vi "write_single_line.vi"(3 "error in (no error)":errorcluster, 4 "First line?":bool, 5 "Data":dbl, 6 "refnum in":refnum<file>) -> (0 "error out":errorcluster, 1 "String":string, 2 "refnum out":refnum<file>)   [LabVIEW 2015]
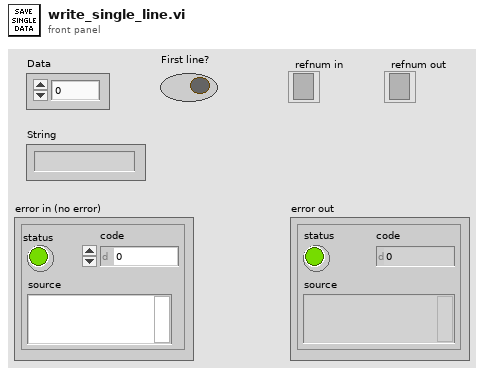
[diagram p1: front panel]
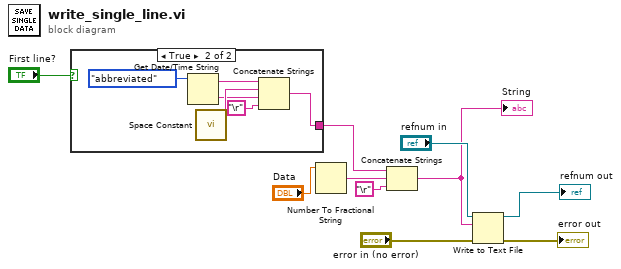
[diagram p0: block diagram]
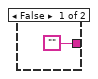
[diagram p2: hidden frame]
diagram:
  n1 = case shown="True" "First line?" {
    tunnel: ["" w12] -> w8
    frame False {
    }
    frame True {
      n2 = Get Date/Time String(date format (0)=enum16{"short", "long", "abbreviated"}."abbreviated") -> (date string=w17:string, time string=w14:string)  [unwired: 2 in]
      n3 = call <vilib>:"Space Constant.vi"() -> ("String"=w15:string)
      n4 = Concatenate Strings(w17, w15, w14, "\r") -> (w12:string)
    }
  }
  n5 = Number To Fractional String(number="Data") -> (F-format string=w7:string)  [unwired: 3 in]
  n6 = Concatenate Strings(w8, w7, "\r") -> (w3:string)
  "String" <- w3
  n7 = Write to Text File(file (use dialog)="refnum in", text=w3, error in="error in (no error)") -> (refnum out=→"refnum out":refnum<file>, error out=→"error out":errorcluster)  [unwired: 1 in, 1 out]
